vi "Read Device Identification Response.vi"(8 "error in":errorcluster, 10 "modbus data unit in":refnum<class "Modbus Data Unit.lvclass">) -> (0 "error out":errorcluster, 2 "Objects":T1[](array[typedef]) {"Object ID" format="%x"}, 4 "Next Object ID":u8, 5 "Conformity Level":T2 items=["None"=0, "Basic Stream"=1, "Regular Stream"=2, "Extended Stream"=3, "Basic Stream/Individual"=129, "Regular Stream/Individual"=130, "Extended Stream/Individual"=131], 6 "done?":bool)   [LabVIEW 2021, in "Master Function Definition.lvclass"]
uses:
  Master Function Definition.lvclass
  Modbus Data Unit/Modbus Data Unit.lvclass
  Data Model/Device ID Type.ctl
  Data Model/Identification Parameters.ctl
  Modbus Data Unit/Modbus Data Unit.lvclass/Modbus Data Unit.ctl
  Modbus Data Unit/Deconstruct PDU.vi
  Master Function Definition.lvclass/Master Function Definition.ctl
  Data Model/Device Data Model.lvclass
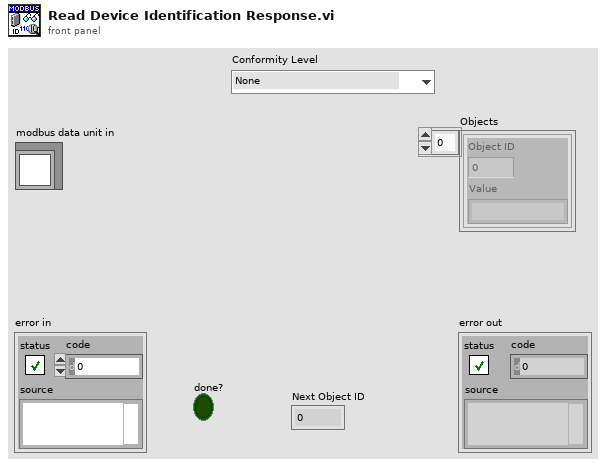
[diagram p1: front panel]
types:
  T1 = typedef "Device Data Model.lvclass/Identification Parameters.ctl" = cluster{"Object ID":u8, "Value":string}
  T2 = typedef "Device Data Model.lvclass/Device ID Type.ctl" = u8
  T3 = typedef "Modbus Data Unit.lvclass/Function.ctl" = u8
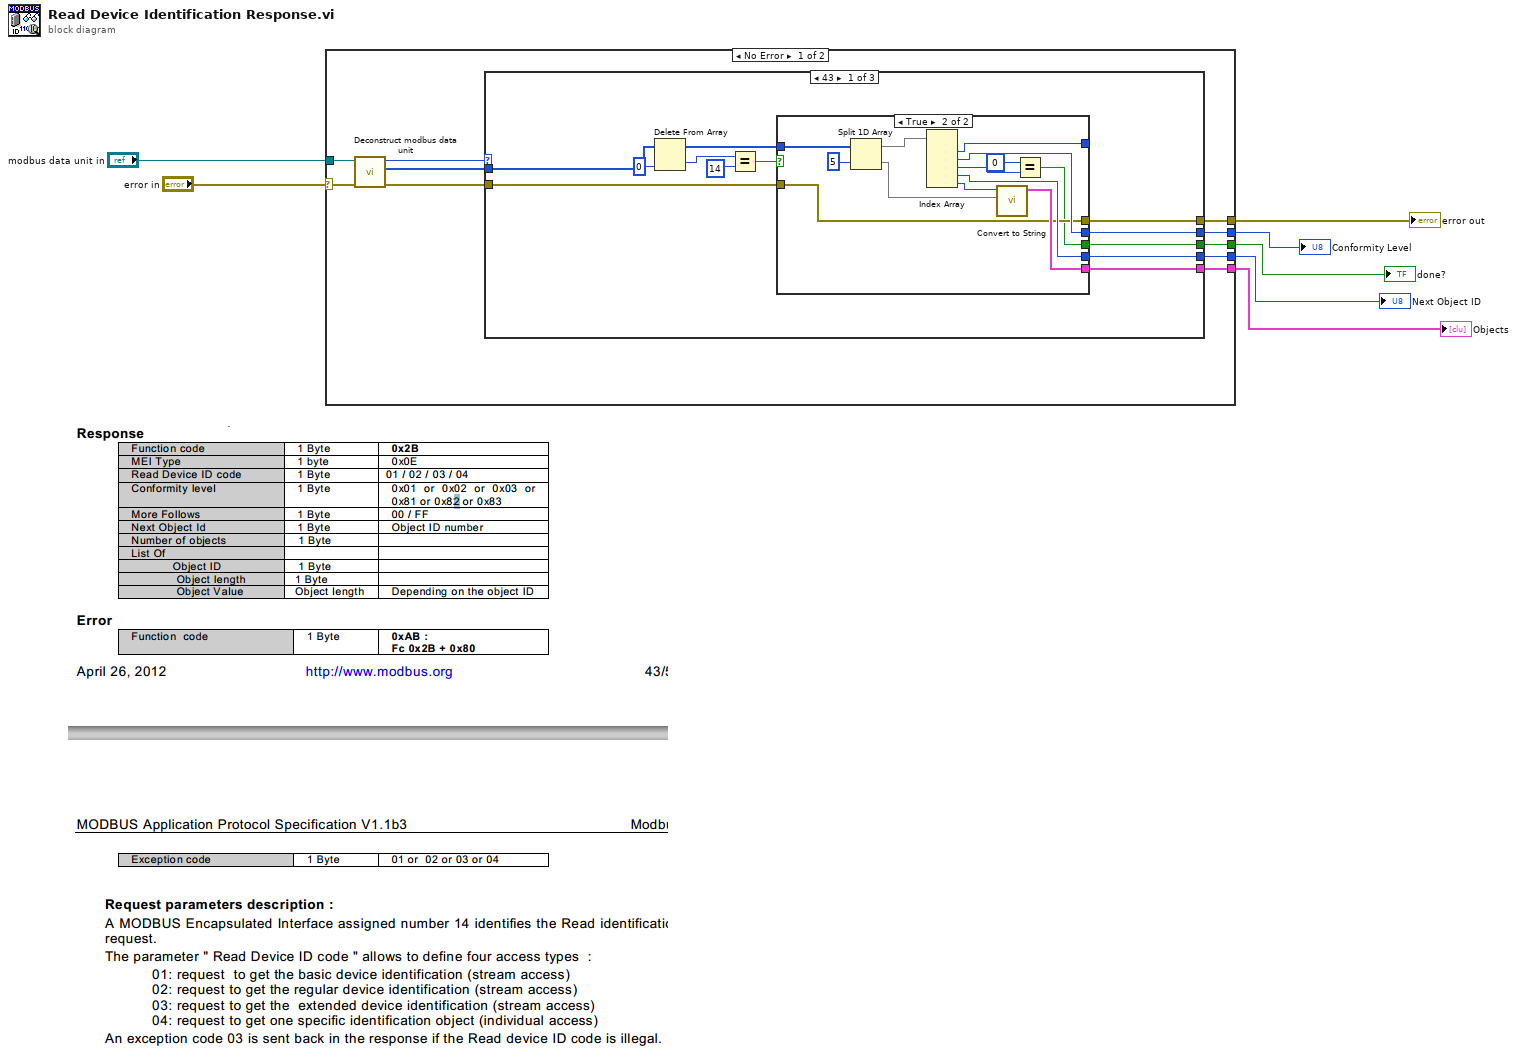
[diagram p0: block diagram]
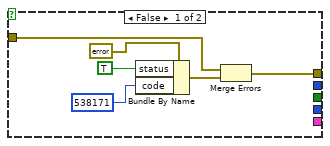
[diagram p2: hidden frame]
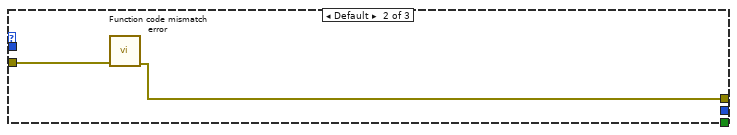
[diagram p3: hidden frame]
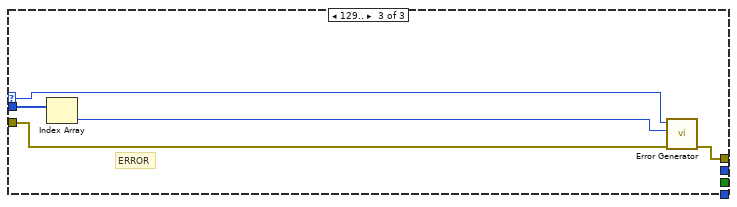
[diagram p4: hidden frame]
diagram:
  n1 = case shown="No Error" "error in" {
    selector: "error in" -> [w16 w56]
    tunnel: [w17 w56] -> w6
    tunnel: "modbus data unit in" -> [w14 _]
    tunnel: [w12 _] -> w3
    tunnel: [w11 _] -> w4
    tunnel: [w10 _] -> w2
    tunnel: [w9 _] -> w1
    frame No Error {
      n2 = call "Deconstruct modbus data unit.vi"("error in"=w16, "modbus data unit in"=w14) -> ("error out"=w13:errorcluster, "data"=w15:u8[], "Function"=w8:T3)  [unwired: 7 in]
      n3 = case shown="43" w8 {
        selector: w8 -> [_ _ w51]
        tunnel: w13 -> [w27 w50 w52]
        tunnel: w15 -> [w29 _ w55]
        tunnel: [w28 w49 w54] -> w17
        tunnel: [w26 _ _] -> w12
        tunnel: [w25 _ _] -> w11
        tunnel: [w24 _ _] -> w10
        tunnel: [w23 _ _] -> w9
        frame 43 {
          n4 = Delete From Array(array=w29, index=0) -> (deleted portion=w21:u8, array with subset deleted=w22:u8[])  [unwired: 1 in]
          n5 = Equal?(x=w21, y=u8 14) -> (x = y?=w19:bool)
          n6 = case shown="True" w19 {
            tunnel: [_ w39] -> w26
            tunnel: [_ w46] -> w25
            tunnel: [_ w45] -> w24
            tunnel: [_ w44] -> w23
            tunnel: w22 -> [_ w43]
            tunnel: w27 -> [w30 w42]
            tunnel: [w31 w42] -> w28
            tunnel: [_ w36] -> _
            frame False {
              n7 = Bundle By Name(cluster=errorcluster {"status"=FALSE, "code"=0, "source"=""} ("error constant"), "status"=TRUE, "code"=538171) -> (w34:errorcluster)
              n8 = Merge Errors(w30, w34) -> (w31:errorcluster)
            }
            frame True {
              n9 = Split 1D Array(array=w43, index=5) -> (first subarray=w47:u8[], second subarray=w38:u8[])
              n10 = Index Array(array=w47) -> (element #1=w36:u8, element #2=w46:u8, element #3=w41:u8, element #4=w45:u8, element #5=w37:u8)  [unwired: 5 in]
              n11 = call "Convert to String.vi"("Byte Array"=w38, "number of objects"=w37) -> ("Objects"=w44:T1[])  [unwired: 9 in]
              n12 = Equal?(x=u8 0, y=w41) -> (x = y?=w39:bool)
            }
          }
        }
        frame Default {
          n13 = call "Function code mismatch error.vi"("error in (no error)"=w50) -> ("error out"=w49:errorcluster)  [unwired: 10 in]
        }
        frame 129.. {
          # "ERROR"
          n14 = Index Array(array=w55) -> (element=w53:u8)  [unwired: 1 in]
          n15 = call "Error Generator.vi"("error in"=w52, "data return (error code)"=w53, "function return"=w51) -> ("error out"=w54:errorcluster)  [unwired: 8 in]
        }
      }
    }
    frame Error {
    }
  }
  "error out" <- w6
  "Conformity Level" <- w4
  "done?" <- w3
  "Next Object ID" <- w2
  "Objects" <- w1
